vi "check item.vi"(0 "string in":string) -> (4 "nested out":string, 6 "is int?":bool, 8 "is list?":bool, 10 "is nested?":bool, 14 "list out":string[](array[string]), 15 "int out":u8)   [LabVIEW 2019]
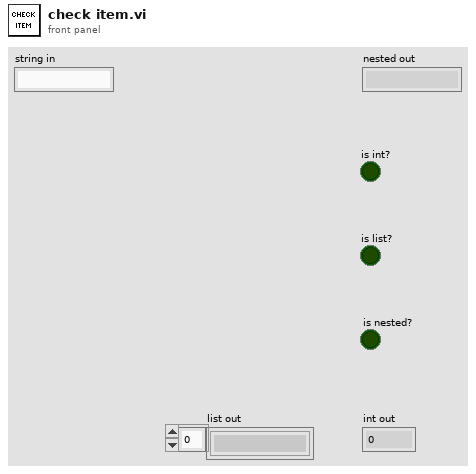
[diagram p1: front panel]
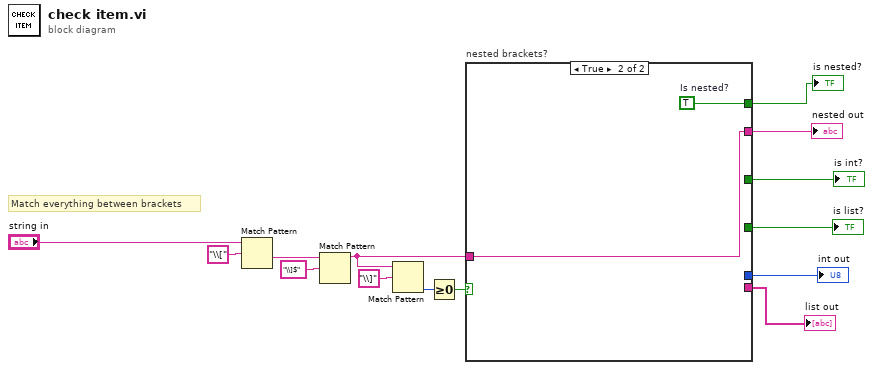
[diagram p0: block diagram]
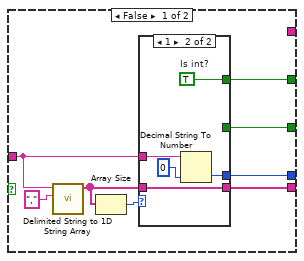
[diagram p2: hidden frame]
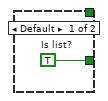
[diagram p3: hidden frame]
diagram:
  # "Match everything between brackets"
  n1 = Match Pattern(string="string in", regular expression="\\[") -> (after substring=w4:string)  [unwired: 1 in, 3 out]
  n2 = Match Pattern(string=w4, regular expression="\\]$") -> (before substring=w7:string)  [unwired: 1 in, 3 out]
  n3 = Match Pattern(string=w7, regular expression="\\]") -> (offset past match=w5:i32)  [unwired: 1 in, 3 out]
  n4 = Greater Or Equal To 0?(x=w5) -> (x >= 0?=w8:bool)
  n5 = case "nested brackets?" shown="True" w8 {
    tunnel: w7 -> [w20 w29]
    tunnel: [_ w30] -> w11
    tunnel: [w18 _] -> w10
    tunnel: [w17 _] -> w9
    tunnel: [_ w29] -> w12
    tunnel: [w16 _] -> w13
    tunnel: [w15 _] -> w14
    frame False {
      n6 = call <vilib>:"Delimited String to 1D String Array.vi"("delimiter"="," ("regular expression"), "delimited string"=w20) -> ("string array"=w19:string[])  [unwired: 9 in]
      n7 = Array Size(array=w19) -> (size(s)=w21:i32)
      n8 = case shown="1" w21 {
        tunnel: w20 -> [_ w26]
        tunnel: w19 -> [_ w27]
        tunnel: [w23 _] -> w18
        tunnel: [_ w28] -> w17
        tunnel: [_ w27] -> w16
        tunnel: [_ w24] -> w15
        frame Default {
          w23 = TRUE  # Is list?
        }
        frame 1 {
          w28 = TRUE  # Is int?
          n9 = Decimal String To Number(string=w26, default (0L)=u8 0) -> (number=w24:u8)  [unwired: 1 in, 1 out]
        }
      }
    }
    frame True {
      w30 = TRUE  # Is nested?
    }
  }
  "is int?" <- w9
  "is list?" <- w10
  "int out" <- w14
  "list out" <- w13
  "nested out" <- w12
  "is nested?" <- w11
